vi "Configure User Defined Event.vi"   [LabVIEW 2021, in "Yokogawa WT1800 Series.lvlib"]
doc: "Configures the user-defined events features.\nUser-defined events can be used to trigger data storage and automatic printing (option)."
uses:
  <instrlib>/Yokogawa WT1800 Series/Yokogawa WT1800 Series.lvlib
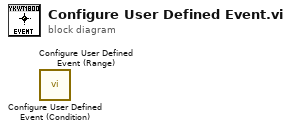
[diagram p0: block diagram]
diagram:
  n1 = call <instrlib>:"Configure User Defined Event (Condition).vi"() -> ()  [unwired: 14 in, 2 out]
  n2 = call <instrlib>:"Configure User Defined Event (Range).vi"() -> ()  [unwired: 14 in, 2 out]
